vi "ZLockRelease.vi"(8 "error in (no error)":errorcluster, 10 "key":string, 11 "ZLock in":refnum<class "ZLock.lvclass">) -> (0 "error out":errorcluster, 2 "key out":string, 3 "ZLock out":refnum<class "ZLock.lvclass">)   [LabVIEW 2010, in "ZLock.lvclass"]
uses:
  <userlib>/bias/subvis/zlock/ZLock.lvclass
  <userlib>/bias/subvis/zlock/ZLock.lvclass/ZLock.ctl
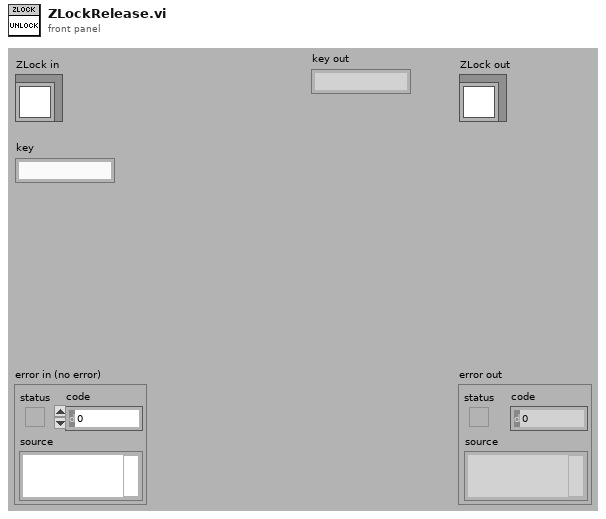
[diagram p1: front panel]
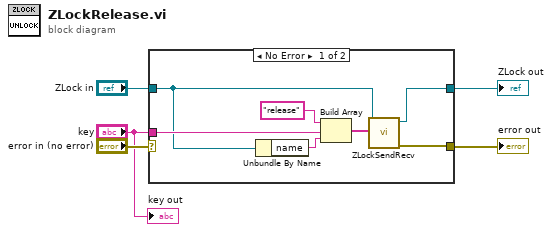
[diagram p0: block diagram]
diagram:
  n1 = case shown="No Error" "error in (no error)" {
    selector: "error in (no error)" -> [_ w14]
    tunnel: [w6 w14] -> w4
    tunnel: [w7 w13] -> w2
    tunnel: "ZLock in" -> [w8 w13]
    tunnel: "key" -> [w10 _]
    frame No Error {
      n2 = Unbundle By Name(w8) -> ("name"=w11:string)
      n3 = Build Array("release" ("data"), w10, w11) -> (w9:string[])
      n4 = call-dynamic "ZLockSendRecv.vi"("parts"=w9, "ZLock in"=w8) -> ("error out"=w6:errorcluster, "ZLock out"=w7:refnum<class "ZLock.lvclass">)  [unwired: 7 in, 1 out]
    }
    frame Error {
    }
  }
  "error out" <- w4
  "ZLock out" <- w2
  "key out" <- "key"
